vi "test.vi"(2 "error in":errorcluster, 3 "Arduino Resource":T1={"VISA resource"="", "Board Type"=enum."Uno", "Connection Type"=enum."USB / Serial", "Bytes Per Packet (15)"=15}, 4 "fb1":u8, 5 "Intensity":u8, 6 "Stress":u8, 7 "Energy":u8) -> (0 "error out 2":errorcluster, 1 "Arduino Resource 2":T1={"VISA resource"="", "Board Type"=enum."Uno", "Connection Type"=enum."USB / Serial", "Bytes Per Packet (15)"=15})   [LabVIEW 2013]
uses:
  <vilib>/LabVIEW Interface for Arduino/Type Defs/Arduino Resource.ctl
  <vilib>/LabVIEW Interface for Arduino/Type Defs/Board Type.ctl
  <vilib>/LabVIEW Interface for Arduino/LabVIEW Interface for Arduino.lvlib
panel:
  in  "fb2":u8
  in  "stop":bool
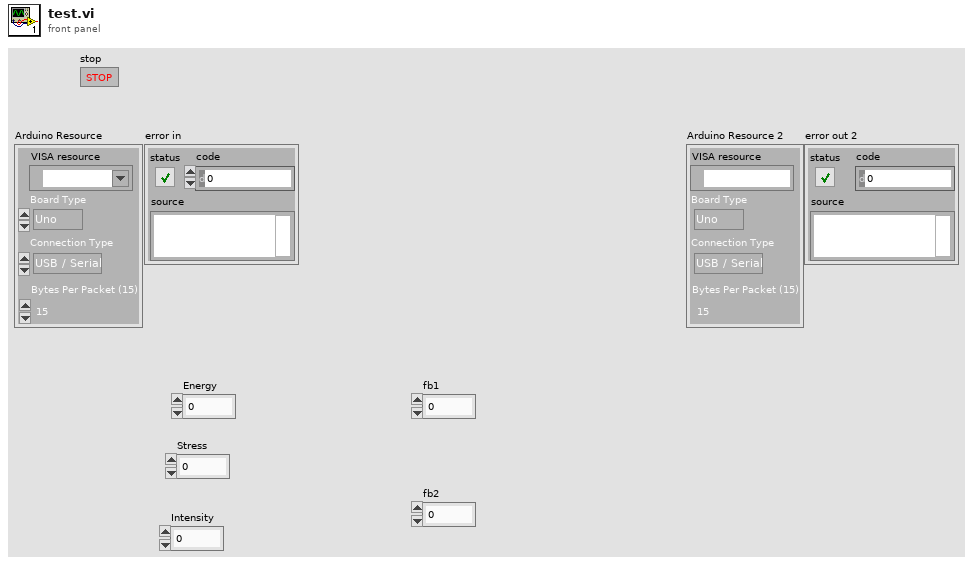
[diagram p1: front panel]
types:
  T1 = typedef "LabVIEW Interface for Arduino.lvlib/Arduino Resource.ctl" = cluster{"VISA resource":refnum<visa-resource-name>, "Board Type":T2, "Connection Type":enum8{"USB / Serial"}, "Bytes Per Packet (15)":u8}
  T2 = typedef "LabVIEW Interface for Arduino.lvlib/Board Type.ctl" = enum16{"Uno", "Dimuelanove w/Atmega 328", "Mega 2560"}
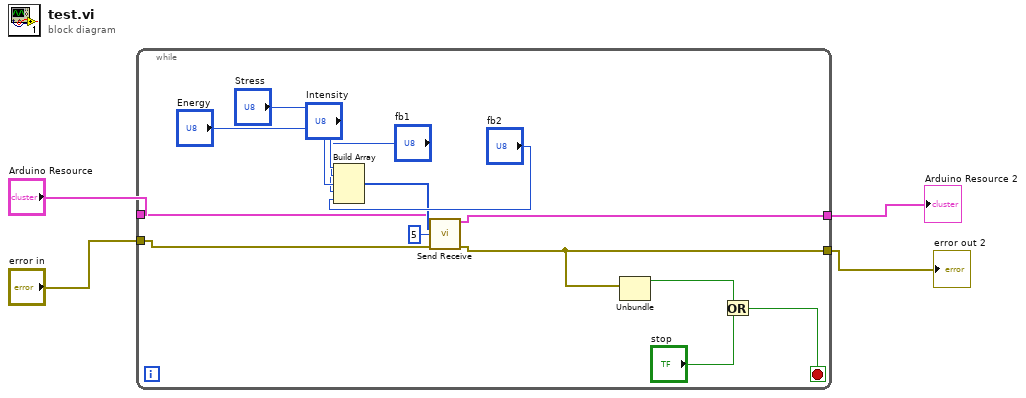
[diagram p0: block diagram]
diagram:
  n1 = while {
    tunnel: "Arduino Resource" -> [w12]
    tunnel: "error in" -> [w11]
    tunnel: [w10] -> w2
    tunnel: [w8] -> w1
    stop <- w5 stop-if-true
    n2 = Build Array("Energy", "Stress", "Intensity", "fb1", "fb2") -> (w13:u8[])
    n3 = call <vilib>:"Send Receive.vi"("Arduino Resource"=w12, "Data"=w13, "Bytes To Read (0)"=u8 5, "error in"=w11) -> ("Arduino Resource"=w10:T1, "error out"=w8:errorcluster)  [unwired: 9 in, 1 out]
    n4 = Unbundle(w8) -> ("status"=w7:bool)  [unwired: 2 out]
    n5 = Or(x=w7, y="stop") -> (x .or. y?=w5:bool)
  }
  "Arduino Resource 2" <- w2
  "error out 2" <- w1
